vi "Line Detector Get Peaks.vi"(6 "Threshold":dbl, 8 "error in (no error)":errorcluster, 9 "Frequency step":dbl, 10 "Signal":cdb[](array[numeric]), 11 "Line Detector Configuration":T1={"Peak width guess"=500.0, "Background removal"=enum."High-pass", "Smoothing"=enum."Low-pass", "Smooth window"=200.0, "Relative threshold"=0.2, "Finder algorithm"=enum."Wavelet", "Bgd window"=50000.0, "Spectrum recorder module name"="Spectrum Recorder", "Fit window"=1000.0, "Initial fit guess"=enum."Peak finder", "Follow\npeaks"=FALSE, "Re-sample"=nan} {"Re-sample" format="%#_6pHz"; "Fit window" format="%#_6pHz"; "Bgd window" format="%#_6pHz"; "Smooth window" format="%#_6pHz"; "Peak width guess" format="%#_6pHz"}) -> (0 "error out":errorcluster, 1 "Peak amplitudes":dbl[](array[numeric]) format="%#_4p", 2 "Peak locations":dbl[](array[numeric]) format="%#_4p")   [LabVIEW 2016]
uses:
  LabActor/Post-Processors/Line Detector/Resonance Detector Configuration.ctl
  <vilib>/addons/Wavelet Analysis/application.llb/WA Multiscale Peak Detection (Array).vi
  <vilib>/Analysis/NI_AAL_SigProc.lvlib
  <vilib>/addons/_Advanced Signal Processing/NI_AdvSigProcWA.lvlib
panel:
  # "F0         dF     Ampl   Phase   Xbgrd   Ybgrd"
  # "Peak finder config"
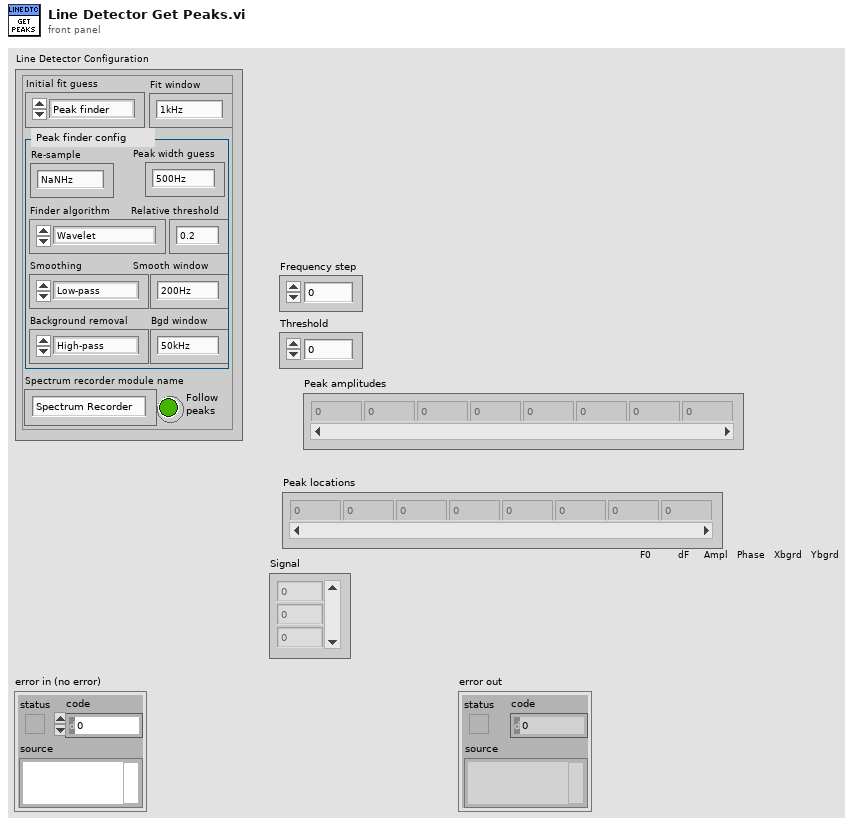
[diagram p1: front panel]
types:
  T1 = typedef "Resonance Detector Configuration.ctl" = cluster{"Peak width guess":dbl, "Background removal":enum16{"NONE", "High-pass", "Detrend"}, "Smoothing":enum16{"NONE", "Low-pass", "Denoise"}, "Smooth window":dbl, "Relative threshold":dbl, "Finder algorithm":enum16{"Basic", "Wavelet", "Wavelet+detrend"}, "Bgd window":dbl, "Spectrum recorder module name":string, "Fit window":dbl, "Initial fit guess":enum16{"Peak finder", "Last fit"}, "Follow\npeaks":bool, "Re-sample":dbl}
  T2 = cluster{"detrend? (F)":bool, "threshold frequency":dbl}
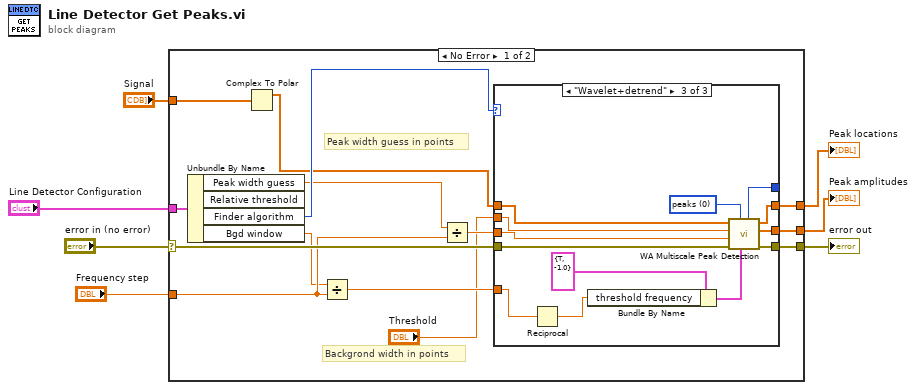
[diagram p0: block diagram]
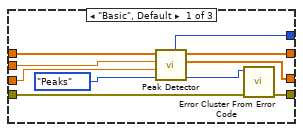
[diagram p2: hidden frame]
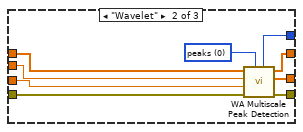
[diagram p3: hidden frame]
diagram:
  n1 = case shown="No Error" "error in (no error)" {
    selector: "error in (no error)" -> [w20 w54]
    tunnel: "Line Detector Configuration" -> [w21 _]
    tunnel: [w18 w54] -> w5
    tunnel: "Signal" -> [w19 _]
    tunnel: "Frequency step" -> [w17 _]
    tunnel: [w10 _] -> w2
    tunnel: [w9 _] -> w1
    frame No Error {
      # "Backgrond width in points"
      # "Peak width guess in points"
      n2 = Unbundle By Name(w21) -> ("Peak width guess"=w15:dbl, "Finder algorithm"=w16:enum16{"Basic", "Wavelet", "Wavelet+detrend"}, "Bgd window"=w13:dbl)  [unwired: 1 out]
      n3 = Complex To Polar(r * e^(i*theta)=w19) -> (r=w11:dbl[])  [unwired: 1 out]
      n4 = Divide(x=w13, y=w17) -> (x/y=w12:dbl)
      n5 = Divide(x=w15, y=w17) -> (x/y=w14:dbl)
      n6 = case shown="\"Wavelet+detrend\"" w16 {
        tunnel: w11 -> [w31 w40 w53]
        tunnel: [w30 w33 w46] -> w9
        tunnel: [w29 w38 w51] -> w10
        tunnel: [w23 w34 w47] -> w18
        tunnel: [w28 w39 w52] -> _
        tunnel: w14 -> [w27 w37 w50]
        tunnel: "Threshold" -> [w26 w36 w49]
        tunnel: w20 -> [w22 w35 w48]
        tunnel: w12 -> [_ _ w41]
        frame "Basic", Default {
          n7 = call <vilib>:"Peak Detector.vi"("peaks/valleys"=enum32{"Peaks", "Valleys"}."Peaks", "width"=w27, "threshold"=w26, "X"=w31) -> ("error"=w24:i32, "Amplitudes"=w30:dbl[], "Locations"=w29:dbl[], "# found"=w28:i32)  [unwired: 3 in, 1 out]
          n8 = call <vilib>:"Error Cluster From Error Code.vi"("error in (no error)"=w22, "error code (0)"=w24) -> ("error out"=w23:errorcluster)  [unwired: 7 in]
        }
        frame "Wavelet" {
          w32 = u16 0 items=["peaks", "valleys"] ("peaks/valleys")
          n9 = call-poly <vilib>:"WA Multiscale Peak Detection.vi"("peaks/valleys"=w32, "error in (no error)"=w35, "width"=w37, "threshold"=w36, "signal"=w40) -> ("error out"=w34:errorcluster, "amplitude"=w33:dbl[], "location"=w38:dbl[], "number of peaks"=w39:i32)  [unwired: 2 in, 1 out]
        }
        frame "Wavelet+detrend" {
          w45 = u16 0 items=["peaks", "valleys"] ("peaks/valleys")
          n10 = Reciprocal(x=w41) -> (1/x=w42:dbl)
          n11 = Bundle By Name(cluster=T2 {"detrend? (F)"=TRUE, "threshold frequency"=-1.0} ("detrend settings"), "threshold frequency"=w42) -> (w43:T2)
          n12 = call-poly <vilib>:"WA Multiscale Peak Detection.vi"("detrend settings"=w43, "peaks/valleys"=w45, "error in (no error)"=w48, "width"=w50, "threshold"=w49, "signal"=w53) -> ("error out"=w47:errorcluster, "amplitude"=w46:dbl[], "location"=w51:dbl[], "number of peaks"=w52:i32)  [unwired: 1 in, 1 out]
        }
      }
    }
    frame Error {
    }
  }
  "error out" <- w5
  "Peak locations" <- w2
  "Peak amplitudes" <- w1
